vi "Write data.vi"(8 "error in (no error)":errorcluster, 10 "data":refnum<class>, 11 "Node in":refnum<class "ListNode.lvclass">) -> (0 "error out":errorcluster, 3 "Node out":refnum<class "ListNode.lvclass">)   [LabVIEW 2010, in "ListNode.lvclass"]
uses:
  ListNode.lvclass
  ListNode.lvclass/ListNode.ctl
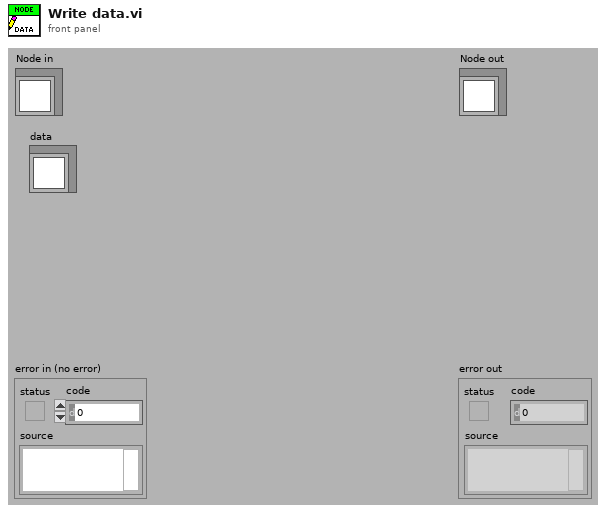
[diagram p1: front panel]
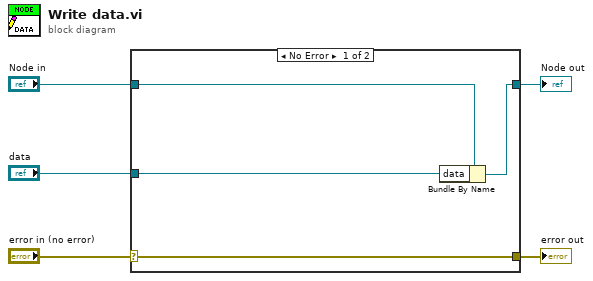
[diagram p0: block diagram]
diagram:
  n1 = case shown="No Error" "error in (no error)" {
    selector: "error in (no error)" -> [w9 w10]
    tunnel: [w9 w10] -> w4
    tunnel: [w7 w11] -> w2
    tunnel: "Node in" -> [w8 w11]
    tunnel: "data" -> [w6 _]
    frame No Error {
      n2 = Bundle By Name(cluster=w8, "data"=w6) -> (w7:refnum<class "ListNode.lvclass">)
    }
    frame Error {
    }
  }
  "error out" <- w4
  "Node out" <- w2
